vi "Main.vi"() -> ()   [LabVIEW 2019]
uses:
  VIs/Telas.ctl
  VIs/TelaParametrosTeste/VariaveisParametros.vi
  VIs/Main/VariaveisTaskMedicao.vi
  Users/Nicole/Downloads/a/ims-desktop/Variaveis/CodOrder.vi
  Users/Nicole/Downloads/a/ims-desktop/Variaveis/User.vi
panel:
  out "String":string
  out "RedimensionarTela":bool
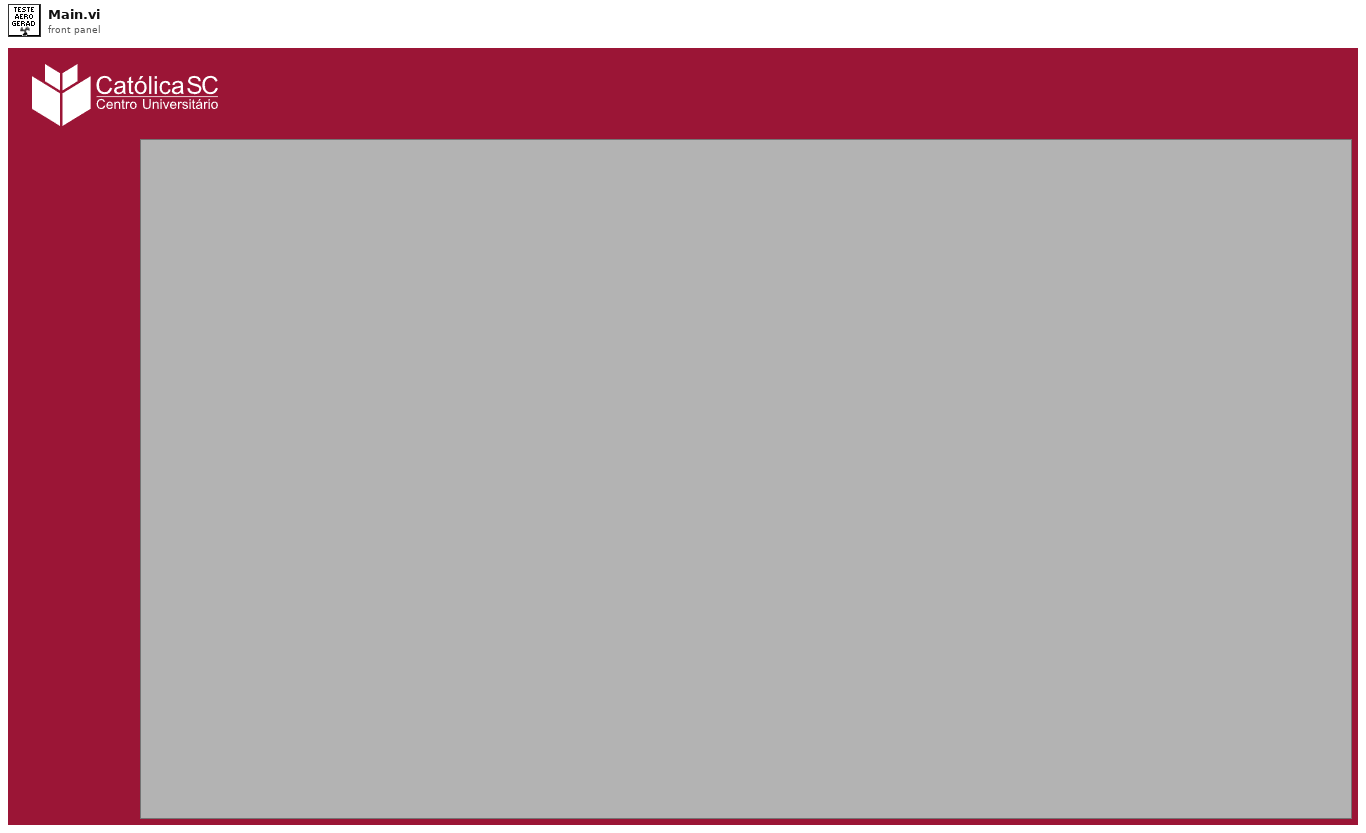
[diagram p1: front panel]
types:
  T1 = enum32{"invalid app kind", "Development System", "Run Time System", "Student Edition", "Embedded LabVIEW", "Evaluation", "Custom"}
  T2 = typedef "Telas.ctl" = enum16{"Operator", "MeasureFrameTestCommunication", "MeasureFrame", "CNCLoadProgram", "RotorBrokenBars", "Configuration", "MeasureFramePreparation", "WindingLabel", "OtherLabel", "InsulationTapeLabel", "WindingSpecialLabel", "GCF", "AssemblyWindingLabel", "Press", "ThermalProtectorLabel", "Traceability", "MeasureFrameProductionOrder", "MeasureFrameStandardEquipment", "MeasureFrameReferentiate", "LabelScanner", "Alerts", "ProductImages", "QGA", "RotorExternalDiameter", "ComponentRegistration", "WindingInspectionInsulationTapeId", "WindingInspectionPreparation", "WindingInspectionMonitoring", "BearingStiffnessMotorIdentification", "BearingStiffnessLvdtSetup", "BearingStiffness", "WindingInspectionMeasureResistance", "BearingStiffnessManualMode", "Calibration", "PressTooling", "GageDrawing", "BalancingReportProductionOrder", "BalancingReport", "PressMeasureAndControl", "WireFaultDetectionMAG", "StatorImpregnationWeight", "MeasureCapacitance", "SpecialCover", "RegistrationOfInspectionDocuments", "BearingHouseDiameter", "HeaterTemperatureRecord", "PackageLength", "Cnc", "BadgeRegistration", "SpecialFrame", "TerminalBoxFitting", "CoordinateMeasuringMachineDataConversion", "Checklist", "FrameCoverFit", "ShaftGrindingInspection", "ShaftBearingPress", "RotorHeatTreatment", "PressingMeasureBeatPulley", "MotorVisualInspection", "VacuumImpregnation", "Standards", "PaintPreparation", "Runout", "RotorPressingDimension"}
  T3 = typedef "Telas.ctl" = enum16{"Selecao", "Config", "Medicao", "ParametrosTeste"}
  T4 = enum16{"NoAccess", "Administrator", "Analyst", "Operator"}
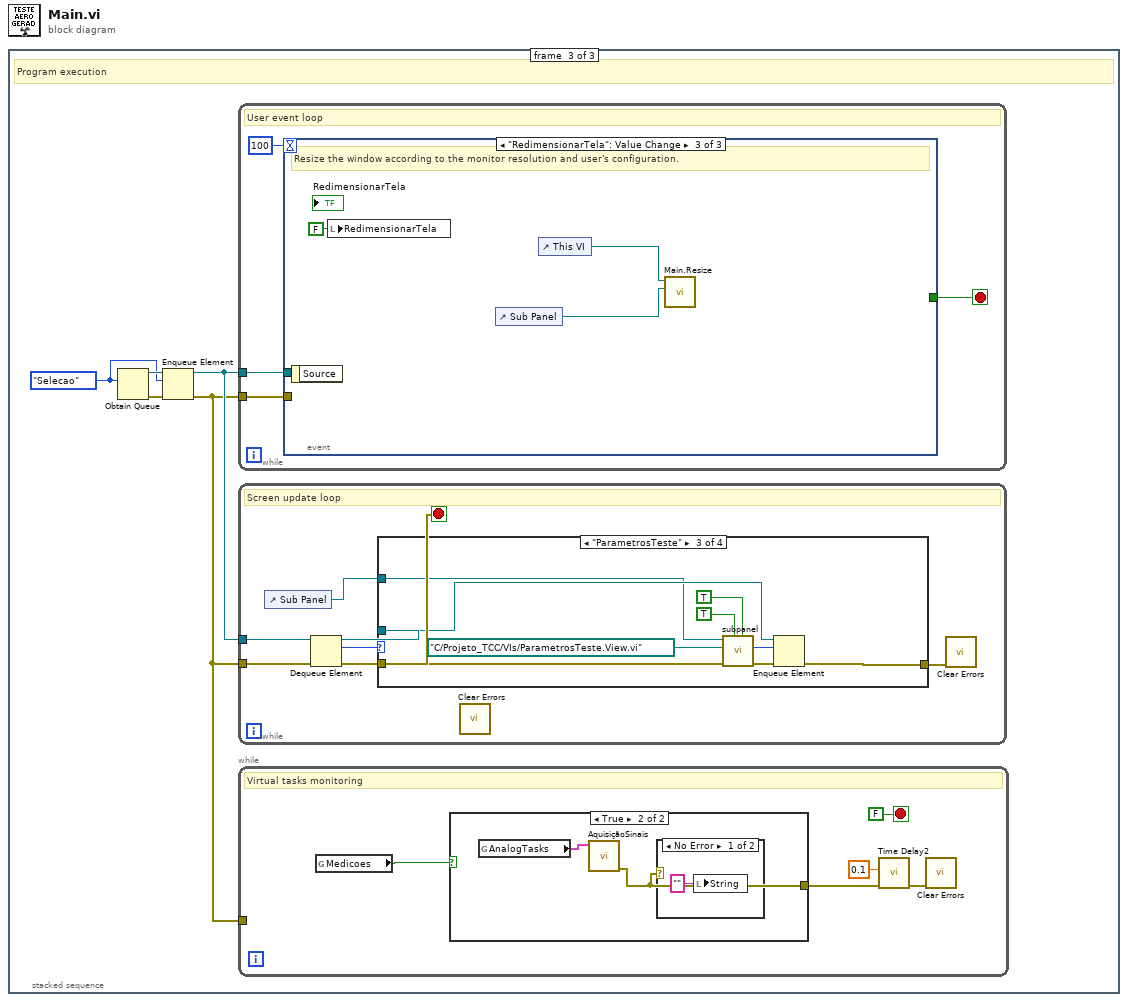
[diagram p0: block diagram]
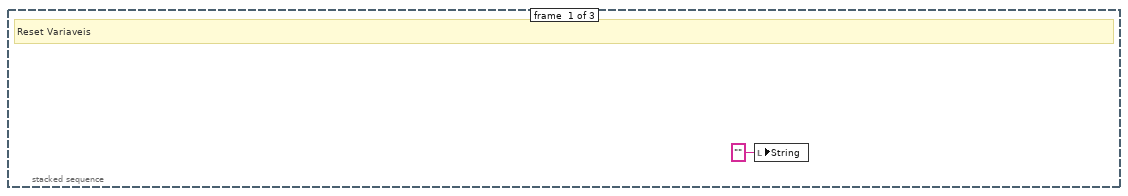
[diagram p2: hidden frame]
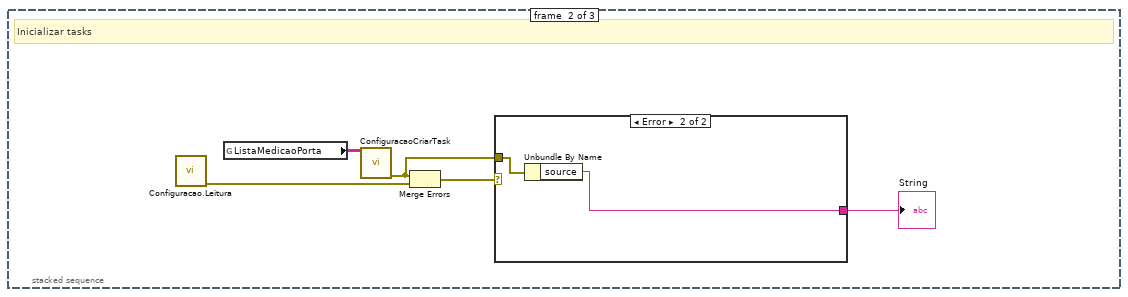
[diagram p3: hidden frame]
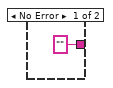
[diagram p4: hidden frame]
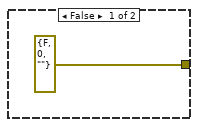
[diagram p5: hidden frame]
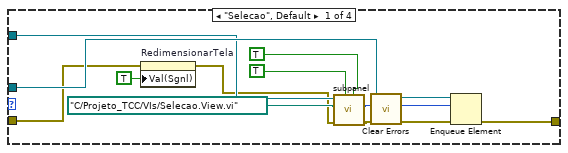
[diagram p7: hidden frame]
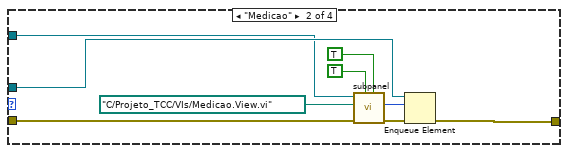
[diagram p8: hidden frame]
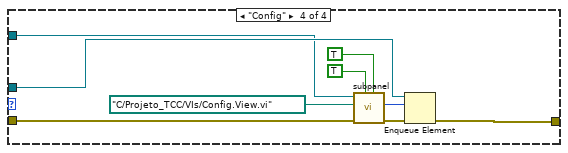
[diagram p9: hidden frame]
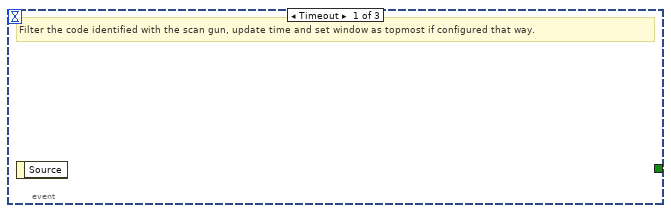
[diagram p10: hidden frame]
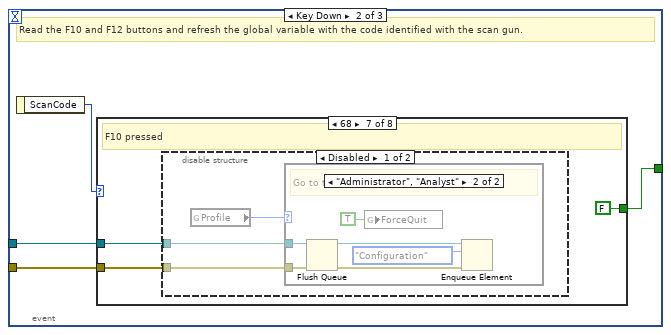
[diagram p11: hidden frame]
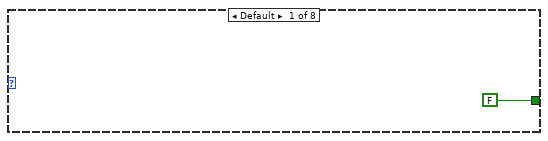
[diagram p12: hidden frame]
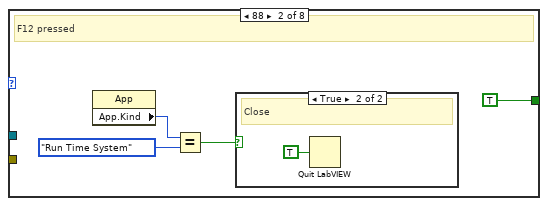
[diagram p13: hidden frame]
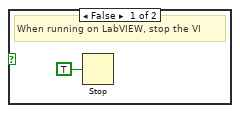
[diagram p14: hidden frame]
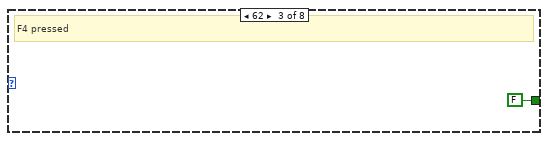
[diagram p15: hidden frame]
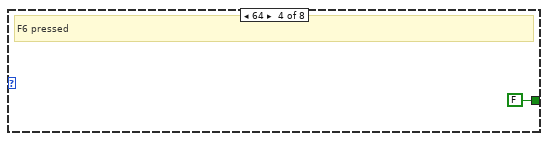
[diagram p16: hidden frame]
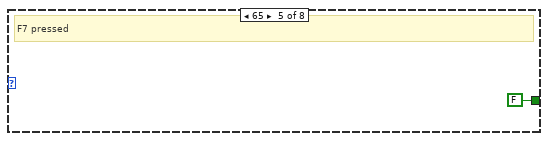
[diagram p17: hidden frame]
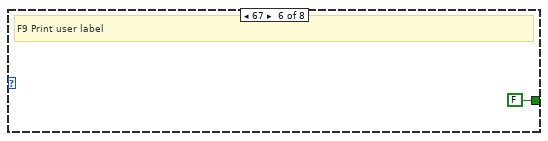
[diagram p18: hidden frame]
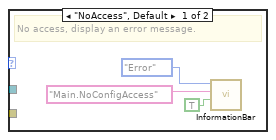
[diagram p19: hidden frame]
diagram:
  n1 = stacked-sequence {
    frame #0 {
      # "Reset Variaveis"
      n2 = local write "String"("" ("String")) -> ()
    }
    frame #1 {
      # "Inicializar tasks"
      n3 = call "Configuracao.Leitura.vi"() -> ("error out"=w5:errorcluster)  [unwired: 11 in]
      n4 = global read "VariaveisParametros.vi" "ListaMedicaoPorta"() -> (w6:string[][])
      n5 = call "ConfiguracaoCriarTask.vi"("ListaMedicaoPorta"=w6) -> ("error out"=w3:errorcluster)  [unwired: 9 in, 1 out]
      n6 = Merge Errors(w3, w5) -> (w4:errorcluster)
      n7 = case shown="Error" w4 {
        tunnel: w3 -> [_ w9]
        tunnel: ["" ("source") w8] -> w2
        frame No Error {
        }
        frame Error {
          n8 = Unbundle By Name(w9) -> ("source"=w8:string)
        }
      }
      "String" <- w2
    }
    frame #2 {
      w12 = Telas."Selecao" ("NextScreen")
      # "Program execution"
      n9 = Obtain Queue(element data type=w12) -> (queue out=w13:refnum<queue>, error out=w14:errorcluster)  [unwired: 4 in, 1 out]
      n10 = Enqueue Element(queue=w13, element=w12, error in (no error)=w14) -> (queue out=w11:refnum<queue>, error out=w10:errorcluster)  [unwired: 1 in, 1 out]
      n11 = while {
        tunnel: w11 -> [w71]
        tunnel: w10 -> [w70]
        stop <- w73 stop-if-true
        # "User event loop"
        n12 = event shown="[2] \"RedimensionarTela\": Value Change" {
          selector: _ -> [_ _ _]
          dyn-events: _ -> [_ _ _]
          timeout: 100 -> [_ _ _]
          tunnel: [_ w76 _] -> w73
          tunnel: w71 -> [_ w74 _]
          tunnel: w70 -> [_ w75 _]
          event Timeout {
            # "Filter the code identified with the scan gun, update time and set window as topmost if configured that way."
            n13 = event-data() -> ()  [unwired: 1 in, 1 out]
          }
          event Key Down {
            # "Read the F10 and F12 buttons and refresh the global variable with the code identified with the scan gun."
            n14 = event-data() -> ("ScanCode"=w77:i16)  [unwired: 1 in]
            n15 = case shown="68" w77 {
              tunnel: [FALSE TRUE FALSE FALSE FALSE FALSE FALSE FALSE] -> w76
              tunnel: w75 -> [_ _ _ _ _ _ w90 _]
              tunnel: w74 -> [_ _ _ _ _ _ w89 _]
              frame Default {
              }
              frame 88 {
                # "F12 pressed"
                n16 = property class="App"() -> ("App.Kind"=w81:T1)  [unwired: 2 in, 2 out]
                n17 = Equal?(x=w81, y=T1."Run Time System") -> (x = y?=w79:bool)
                n18 = case shown="True" w79 {
                  frame False {
                    # "When running on LabVIEW, stop the VI"
                    n19 = Stop(stop? (T)=TRUE) -> ()
                  }
                  frame True {
                    # "Close"
                    n20 = Quit LabVIEW(quit? (T)=TRUE) -> ()
                  }
                }
              }
              frame 62 {
                # "F4 pressed"
              }
              frame 64 {
                # "F6 pressed"
              }
              frame 65 {
                # "F7 pressed"
              }
              frame 67 {
                # "F9 Print user label"
              }
              frame 68 {
                # "F10 pressed"
                n21 = disable-structure shown="Disabled" {
                  disable-tunnel: w90 -> [w94 _]
                  disable-tunnel: w89 -> [w93 _]
                  frame Disabled {
                    n22 = global read "User.vi" "Profile"() -> (w92:T4)
                    n23 = case shown="\"Administrator\", \"Analyst\"" w92 {
                      tunnel: w94 -> [_ w100]
                      tunnel: w93 -> [_ w99]
                      frame "NoAccess", Default {
                        # "No access, display an error message."
                        n24 = call "InformationBar.vi"("BlinkAlert"=TRUE, "Message"="Main.NoConfigAccess", "AlertType"=enum16{"Error", "Warning", "Ok", "Time"}."Error") -> ()  [unwired: 8 in, 1 out]
                      }
                      frame "Administrator", "Analyst" {
                        # "Go to the Configuration Screen."
                        n25 = Flush Queue(queue=w99, error in (no error)=w100) -> (queue out=w102:refnum<queue>, error out=w103:errorcluster)  [unwired: 1 out]
                        n26 = global write "CodOrder.vi" "ForceQuit"(TRUE ("ForceQuit")) -> ()
                        n27 = Enqueue Element(queue=w102, element=Telas."Configuration", error in (no error)=w103) -> ()  [unwired: 1 in, 3 out]
                      }
                    }
                  }
                  frame Enabled {
                  }
                }
              }
              frame 87 {
                # "F11 pressed"
              }
            }
          }
          event "RedimensionarTela": Value Change {
            # "Resize the window according to the monitor resolution and user's configuration."
            n28 = event-data() -> ()  [unwired: 1 in, 1 out]
            n29 = local write "RedimensionarTela"(FALSE ("Resize")) -> ()
            n30 = control-ref of="Sub Panel"() -> (w105:refnum<vi>)
            n31 = control-ref of="This VI"() -> (w106:refnum<vi>)
            n32 = call "Main.Resize.vi"("Sub Panel"=w105, "VI in"=w106) -> ()  [unwired: 10 in]
          }
        }
      }
      n33 = while {
        tunnel: w10 -> [w30]
        tunnel: w11 -> [w29]
        stop <- w28 stop-if-true
        # "Screen update loop"
        n34 = control-ref of="Sub Panel"() -> (w24:refnum<vi>)
        n35 = Dequeue Element(queue=w29, error in (no error)=w30) -> (queue out=w27:refnum<queue>, element=w26:T3, error out=w28:errorcluster)  [unwired: 1 in, 1 out]
        n36 = case shown="\"ParametrosTeste\"" w26 {
          tunnel: w27 -> [w42 w46 w55 w64]
          tunnel: w28 -> [w32 w45 w54 w63]
          tunnel: w24 -> [w35 w44 w53 w62]
          tunnel: [w41 w43 w52 w61] -> w25
          frame "Selecao", Default {
            n37 = property on="RedimensionarTela" class="Bool (strict)"(error in=w32, "Val(Sgnl)"=TRUE ("Value (Signaling)")) -> (error out=w31:errorcluster)  [unwired: 1 in, 1 out]
            n38 = call "subpanel.vi"("Panel Transparent"=TRUE, "Wait Until Done"=TRUE, "error in"=w31, "Vi"=path "C:/Projeto_TCC/VIs/Selecao.View.vi", "SubPanel"=w35) -> ("error out"=w40:errorcluster, "NextScreen"=w39:T3)  [unwired: 4 in, 1 out]
            n39 = call <vilib>:"Clear Errors.vi"("error in (no error)"=w40) -> ("error out"=w34:errorcluster)  [unwired: 5 in, 1 out]
            n40 = Enqueue Element(queue=w42, element=w39, error in (no error)=w34) -> (error out=w41:errorcluster)  [unwired: 1 in, 2 out]
          }
          frame "Medicao" {
            n41 = call "subpanel.vi"("Panel Transparent"=TRUE, "Wait Until Done"=TRUE, "error in"=w45, "Vi"=path "C:/Projeto_TCC/VIs/Medicao.View.vi", "SubPanel"=w44) -> ("error out"=w50:errorcluster, "NextScreen"=w51:T3)  [unwired: 4 in, 1 out]
            n42 = Enqueue Element(queue=w46, element=w51, error in (no error)=w50) -> (error out=w43:errorcluster)  [unwired: 1 in, 2 out]
          }
          frame "ParametrosTeste" {
            n43 = call "subpanel.vi"("Panel Transparent"=TRUE, "Wait Until Done"=TRUE, "error in"=w54, "Vi"=path "C:/Projeto_TCC/VIs/ParametrosTeste.View.vi", "SubPanel"=w53) -> ("error out"=w59:errorcluster, "NextScreen"=w60:T3)  [unwired: 4 in, 1 out]
            n44 = Enqueue Element(queue=w55, element=w60, error in (no error)=w59) -> (error out=w52:errorcluster)  [unwired: 1 in, 2 out]
          }
          frame "Config" {
            n45 = call "subpanel.vi"("Panel Transparent"=TRUE, "Wait Until Done"=TRUE, "error in"=w63, "Vi"=path "C:/Projeto_TCC/VIs/Config.View.vi", "SubPanel"=w62) -> ("error out"=w68:errorcluster, "NextScreen"=w69:T3)  [unwired: 4 in, 1 out]
            n46 = Enqueue Element(queue=w64, element=w69, error in (no error)=w68) -> (error out=w61:errorcluster)  [unwired: 1 in, 2 out]
          }
        }
        n47 = call <vilib>:"Clear Errors.vi"() -> ()  [unwired: 6 in, 2 out]
        n48 = call <vilib>:"Clear Errors.vi"("error in (no error)"=w25) -> ()  [unwired: 5 in, 2 out]
      }
      n49 = while {
        tunnel: w10 -> [_]
        stop <- FALSE stop-if-true
        # "Virtual tasks monitoring"
        n50 = global read "VariaveisTaskMedicao.vi" "Medicoes"() -> (w18:bool)
        n51 = case shown="True" w18 {
          tunnel: [errorcluster {"status"=FALSE, "code"=0, "source"=""} ("error out") w21] -> w15
          frame False {
          }
          frame True {
            n52 = global read "VariaveisTaskMedicao.vi" "AnalogTasks"() -> (w22:cluster{"Function":i32, "Task":refnum<k21>}[])
            n53 = call "AquisiçãoSinais.vi"("Analog"=w22) -> ("error out"=w21:errorcluster)  [unwired: 10 in]
            n54 = case shown="No Error" w21 {
              frame No Error {
                n55 = local write "String"("" ("String")) -> ()
              }
              frame Error {
              }
            }
          }
        }
        n56 = call "Time Delay2"("error in (no error)"=w15, "Delay Time (s)"=0.1) -> ("error out"=w16:errorcluster)  [unwired: 9 in]
        n57 = call <vilib>:"Clear Errors.vi"("error in (no error)"=w16) -> ()  [unwired: 5 in, 2 out]
      }
    }
  }
